vi "Shared Instance FGV.vi"(7 "Read?":bool, 11 "LogReference Instance":refnum<class "LoggerReference.lvclass">) -> (3 "Shared Instances":refnum<class "LoggerReference.lvclass">[](array[class]))   [LabVIEW 2020, in "MVA Framework.lvlib" / "Singleton Event Log.lvlib"]
doc: "--\nCopyright © 2017 Composed SystemsI All rights reserved.\n\nAuthor: Jon McBee <jon.mcbee@composed.io>\n\nThis library is provided \"AS IS\" ,WITHOUT WARRANTIES OR\nCONDITIONS OF ANY KIND, either express or implied.\n\nComposed Systems -- composed.io\n\nStream 0.0.1.1\nJon McBee - Composed Systems\nCopyright (c) 2017, Composed Systems"
uses:
  Singleton Event Log.lvlib
  LoggerReference/LoggerReference.lvclass
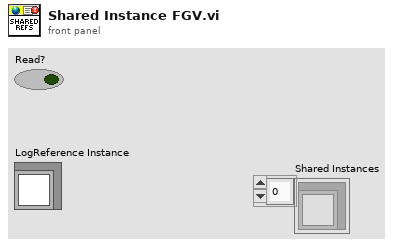
[diagram p1: front panel]
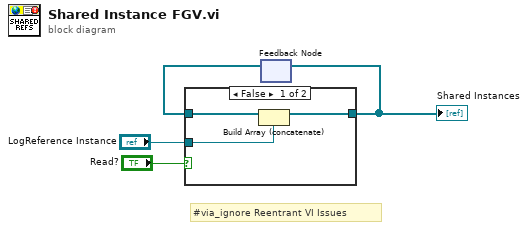
[diagram p0: block diagram]
diagram:
  # "#via_ignore Reentrant VI Issues"
  n1 = feedback #1() -> (w3:refnum<class "LoggerReference.lvclass">[])  [unwired: 1 in]
  n2 = case shown="False" "Read?" {
    tunnel: "LogReference Instance" -> [w5 _]
    tunnel: w3 -> [w7 w8]
    tunnel: [w6 w8] -> w2
    frame False {
      n3 = Build Array (concatenate)(w7, w5) -> (w6:refnum<class "LoggerReference.lvclass">[])
    }
    frame True {
    }
  }
  "Shared Instances" <- w2
  n4 = feedback-in #1(w2) -> ()
